vi "Read Questionable Bit Condition Status.vi"(8 "error in (no error)":errorcluster, 9 "Bit (9)":u8=9 min=9 max=12, 10 "Platform Slot Number (10)":i16=10 min=-1 max=255, 11 "VISA resource name":refnum<visa-resource-name>) -> (0 "error out":errorcluster, 2 "Questionable Condition":i32, 3 "VISA resource name out":refnum<visa-resource-name>)   [LabVIEW 2018, in "LTB-1.lvlib" / "3150.lvlib"]
doc: "Queries the state of a specific bit in QUEStionable regtister set. The bit number indicates for which bit the information must be retrieved in the STATus:QUEStionable status register."
uses:
  3150.lvlib
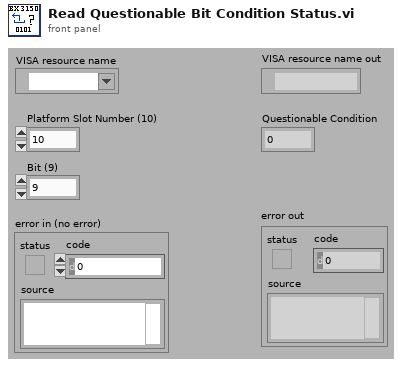
[diagram p1: front panel]
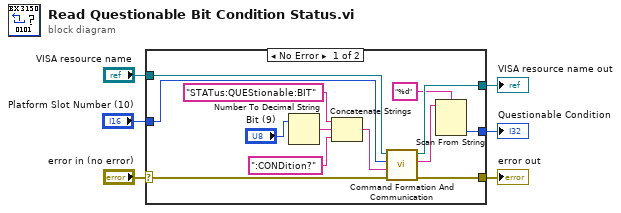
[diagram p0: block diagram]
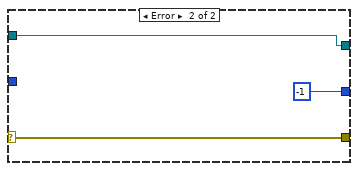
[diagram p2: hidden frame]
diagram:
  n1 = case shown="No Error" "error in (no error)" {
    selector: "error in (no error)" -> [w18 w21]
    tunnel: "VISA resource name" -> [w19 w22]
    tunnel: [w17 w22] -> w4
    tunnel: [w16 w21] -> w3
    tunnel: "Platform Slot Number (10)" -> [w10 _]
    tunnel: [w7 -1] -> w1
    frame No Error {
      n2 = Number To Decimal String(number="Bit (9)") -> (decimal integer string=w13:string)  [unwired: 1 out]
      n3 = Concatenate Strings("STATus:QUEStionable:BIT" ("Command"), w13, ":CONDition?" ("string")) -> (w15:string)
      n4 = call "Command Formation And Communication.vi"("error in (no error)"=w18, "Command"=w15, "Platform Slot Number"=w10, "VISA resource name"=w19) -> ("error out"=w16:errorcluster, "Response"=w8:string, "VISA resource name out"=w17:refnum<visa-resource-name>)  [unwired: 1 in, 4 out]
      n5 = Scan From String(format string="%d", input string=w8) -> (output 1=w7:i32)  [unwired: 2 in, 4 out]
    }
    frame Error {
    }
  }
  "VISA resource name out" <- w4
  "error out" <- w3
  "Questionable Condition" <- w1
